vi "getImage_action.vi"(0 "HGF_IMAQDevice":refnum<class "HGF_IMAQDevice.lvclass">, 2 "Image In":T1, 3 "Buffer Number":u32, 4 "Timeout (1000ms)":i32=1000, 5 "error in (no error)":errorcluster, 6 "Region of Interest":i32[](array[numeric]), 8 "Buffer Number Mode (Next)":T2) -> (11 "Frame Numbers":i32[](array[numeric]), 13 "Image Array":T1[](array[typedef]), 14 "dup HGF_IMAQDevice":refnum<class "HGF_IMAQDevice.lvclass">, 16 "Image Out":T1, 17 "Buffer Number Copied":i32, 18 "Buffer Index Copied":i32, 19 "error out":errorcluster)   [LabVIEW 2014, in "HGF_IMAQ.lvlib" / "HGF_IMAQDevice.lvclass"]
doc: "Returns a copy of an acquired image. IMAQ Copy Acquired Buffer allows you to copy an image from onboard memory to system memory, or from driver-allocated system memory to user-allocated system memory.\n\nCall this VI only after calling IMAQdx Configure Acquisition.vi. If the image type does not match the video format of the camera, this VI changes the image type to a suitable format, at least for IMAQdx."
uses:
  HGF_IMAQDevice.lvclass
  HGF_Auxiliary/HGF_Auxiliary.lvlib
  HGF_Auxiliary/Severity.ctl
  HGF_Auxiliary/ErrorCode.ctl
  <vilib>/vision/Image Controls.llb/IMAQ Image.ctl
  <vilib>/vision/driver/IMAQdx.llb/IMAQdx Buffer Number Mode.ctl
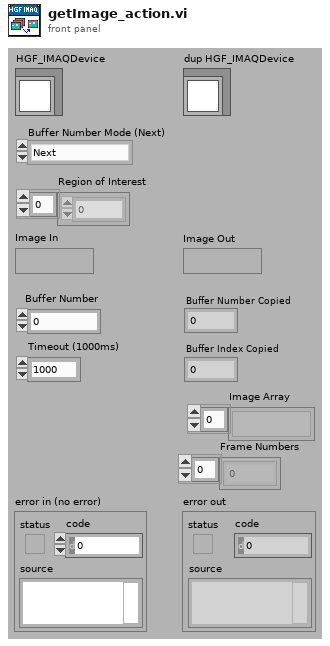
[diagram p1: front panel]
types:
  T1 = typedef "IMAQ Image.ctl" = refnum<image>
  T2 = typedef "NI_Vision_Acquisition_Software.lvlib/IMAQdx Buffer Number Mode.ctl" = enum32{"Next", "Last", "Buffer Number"}
  T3 = typedef "HGF_Auxiliary.lvlib/ErrorCode.ctl" = enum32{"No error", "Function not supported.", "This VI is for friends only.", "Reference object aready exisits.", "Parameter out of range.", "Not a rendezvous.", "Invalid notifier reference.", "Invalid queue reference.", "Self-Test not supported.", "Reset not supported.", "IDN query not supported.", "Error query not supported.", "Incorrect addressee.", "Object already exists.", "No class name specified", "Driver not supported", "Attribute is not writable"}
  T4 = typedef "HGF_Auxiliary.lvlib/Severity.ctl" = enum16{"Info", "Warning", "Fault", "Error", "Fatal"}
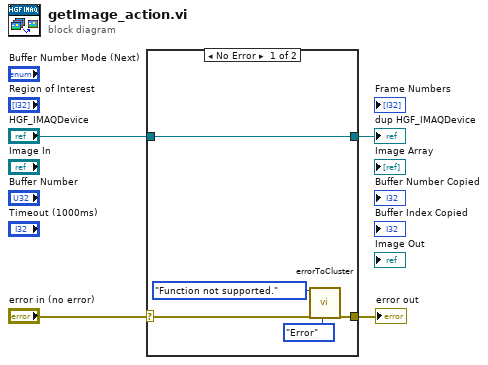
[diagram p0: block diagram]
diagram:
  n1 = case shown="No Error" "error in (no error)" {
    selector: "error in (no error)" -> [w5 w11]
    tunnel: [w6 w11] -> w3
    tunnel: [w9 w10] -> w1
    tunnel: "HGF_IMAQDevice" -> [w9 w10]
    frame No Error {
      n2 = call "errorToCluster.vi"("error code"=ErrorCode."Function not supported.", "error in (no error)"=w5, "severity (Error)"=Severity."Error") -> ("error out"=w6:errorcluster)  [unwired: 2 in, 14 out]
    }
    frame Error {
    }
  }
  "error out" <- w3
  "dup HGF_IMAQDevice" <- w1
